vi "Prompt.vi"(4 "Positive Button (\"Yes\")":string="Yes", 6 "Negative Button (\"No\")":string="No", 8 "error in (no error)":errorcluster, 10 "Prompt":string, 11 "Monitor Test in":refnum<class "Monitor Test.lvclass">) -> (0 "error out":errorcluster, 3 "Monitor Test out":refnum<class "Monitor Test.lvclass">)   [LabVIEW 2017, in "Monitor Test.lvclass"]
uses:
  Monitor Test.lvclass
panel:
  in  "Negative":bool
  in  "Positive":bool
  out "Prompt":string
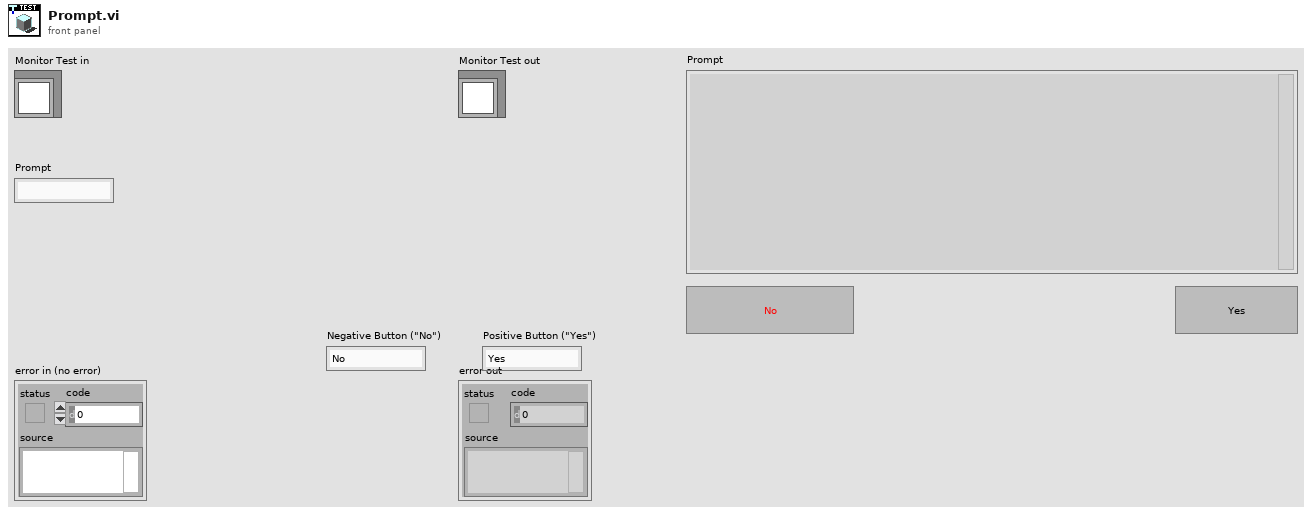
[diagram p1: front panel]
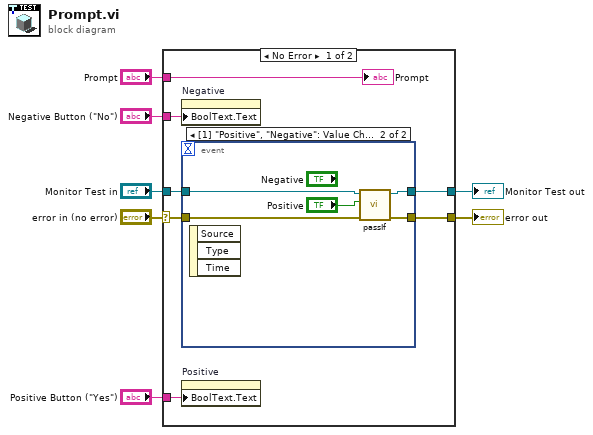
[diagram p0: block diagram]
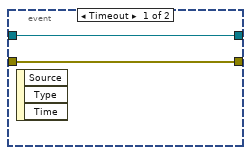
[diagram p2: hidden frame]
diagram:
  n1 = case shown="No Error" "error in (no error)" {
    selector: "error in (no error)" -> [w9 w23]
    tunnel: [w8 w23] -> w6
    tunnel: [w11 w22] -> w4
    tunnel: "Monitor Test in" -> [w10 w22]
    tunnel: "Prompt" -> [w14 _]
    tunnel: "Negative Button (\"No\")" -> [w13 _]
    tunnel: "Positive Button (\"Yes\")" -> [w12 _]
    frame No Error {
      n2 = property on="Negative" class="Bool"("BoolText.Text"=w13) -> ()  [unwired: 2 in, 2 out]
      n3 = event shown="[1] \"Positive\", \"Negative\": Value Change;  Panel Close" {
        selector: _ -> [_ _]
        dyn-events: _ -> [_ _]
        timeout: _ -> [_ _]
        tunnel: [w16 w20] -> w11
        tunnel: w10 -> [w16 w21]
        tunnel: w9 -> [w15 w18]
        tunnel: [w15 w17] -> w8
        event Timeout {
          n4 = event-data() -> ()  [unwired: 1 in, 3 out]
        }
        event "Positive", "Negative": Value Change; Panel Close {
          n5 = event-data() -> ()  [unwired: 1 in, 3 out]
          n6 = call-dynamic "passIf.vi"("error in (no error)"=w18, "pass"="Positive", "TestCase in"=w21) -> ("error out"=w17:errorcluster, "TestCase out"=w20:refnum<class "Monitor Test.lvclass">)  [unwired: 7 in]
        }
      }
      n7 = property on="Positive" class="Bool"("BoolText.Text"=w12) -> ()  [unwired: 2 in, 2 out]
      "Prompt" <- w14
    }
    frame Error {
    }
  }
  "error out" <- w6
  "Monitor Test out" <- w4
